vi "GPIBtest.vi"() -> ()   [LabVIEW 2012]
panel:
  out "错误输出":errorcluster
  out "Read Buffer":string caption="读取缓冲区"
  in  "VISA资源名称":refnum<visa-resource-name>="GPIB0::17::INSTR"
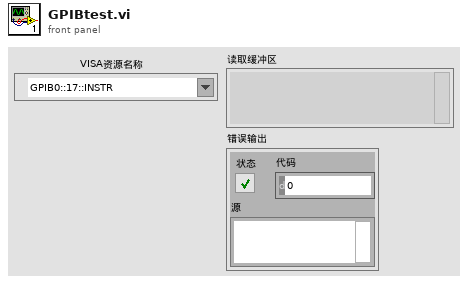
[diagram p1: front panel]
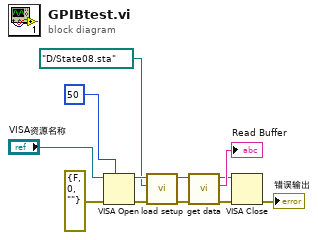
[diagram p0: block diagram]
diagram:
  n1 = VISA Open(timeout (0)=u32 50 ("VISA打开超时（0）"), error in (no error)=errorcluster {"status"=FALSE, "code"=0, "source"=""} ("错误输入（无错误）"), VISA resource name="VISA资源名称") -> (VISA resource name=w9:refnum<visa-resource-name>, error out=w8:errorcluster)  [unwired: 2 in]
  n2 = call "load setup.vi"("错误输入（无错误）"=w8, "path"=path "D:/State08.sta" ("路径"), "VISA GPIB Resource"=w9) -> ("错误输出"=w5:errorcluster, "VISA资源名称输出"=w6:refnum<visa-resource-name>)  [unwired: 7 in]
  n3 = call "get data.vi"("错误输入（无错误）"=w5, "VISA GPIB Resource"=w6) -> ("错误输出"=w2:errorcluster, "Read Buffer"=→"Read Buffer":string, "VISA资源名称输出"=w3:refnum<visa-resource-name>)  [unwired: 6 in, 1 out]
  n4 = VISA Close(VISA resource name=w3, error in (no error)=w2) -> (error out=→"错误输出":errorcluster)
